vi "Perform Measurements.vi"(8 "error in":errorcluster, 9 "Measurement Context":refnum<class "Measure Call Context.lvclass">, 10 "Nominal output voltage":dbl, 11 "Reference values":T2) -> (0 "error out":errorcluster, 1 "Measurement Results":T1, 2 "Load out":refnum<k15>, 3 "Source out":refnum<k15>)   [LabVIEW 2021, in "Line Regulation_PMIC.lvlib"]
uses:
  Line Regulation_PMIC.lvlib
  Measurement Results.ctl
  <vilib>/Plug-In SDKs/Measurements/Measure Call Context/Measure Call Context.lvclass
  <vilib>/Plug-In SDKs/Measurements/Measure Call Context/Accessor/Is Canceled.vi
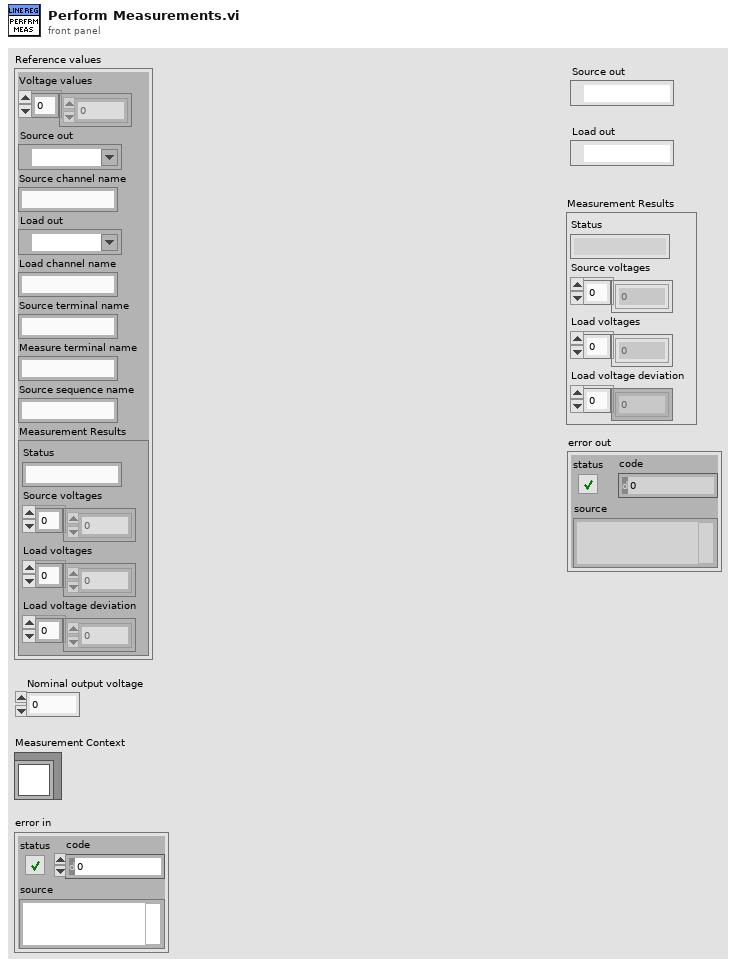
[diagram p1: front panel]
types:
  T1 = typedef "Line Regulation_PMIC.lvlib/Measurement Results.ctl" = cluster{"Status":string, "Source voltages":dbl[], "Load voltages":dbl[], "Load voltage deviation":dbl[]}
  T2 = cluster{"Voltage values":dbl[], "Source out":refnum<k15>, "Source channel name":string, "Load out":refnum<k15>, "Load channel name":string, "Source terminal name":string, "Measure terminal name":string, "Source sequence name":string, "Measurement Results":T1}
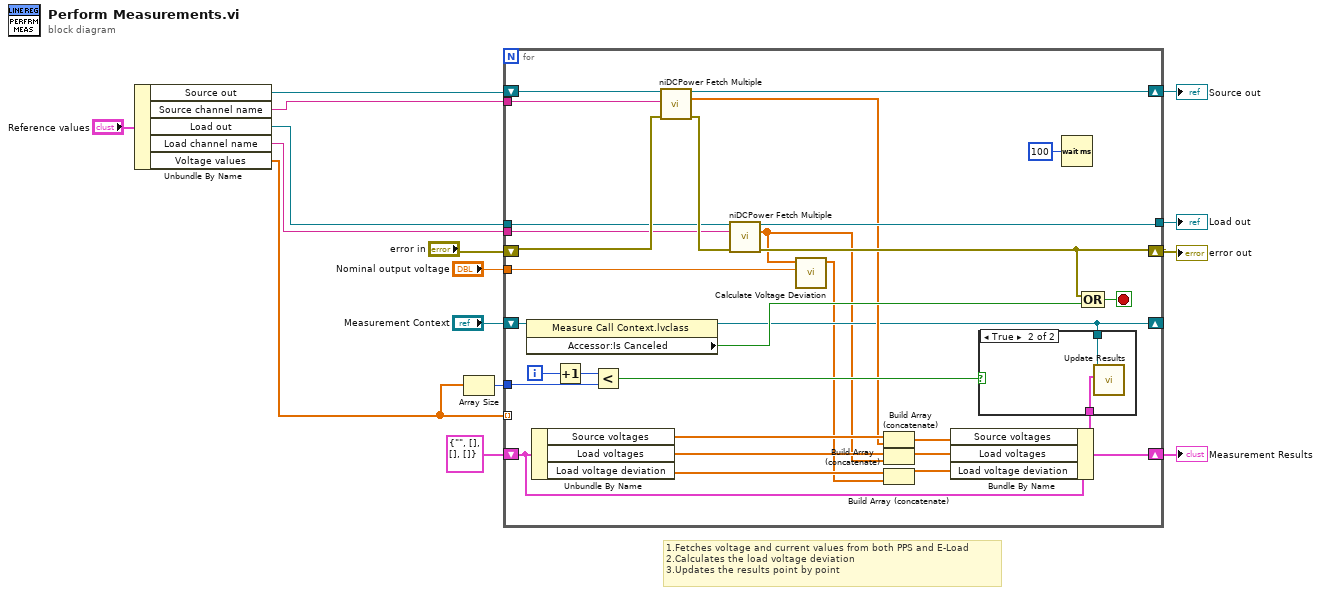
[diagram p0: block diagram]
diagram:
  # "1.Fetches voltage and current values from both PPS and E-Load\n2.Calculates the load voltage deviation\n3.Updates the results point by point"
  n1 = Unbundle By Name("Reference values") -> ("Source out"=w11:refnum<k15>, "Source channel name"=w10:string, "Load out"=w9:refnum<k15>, "Load channel name"=w8:string, "Voltage values"=w6:dbl[])
  n2 = Array Size(array=w6) -> (size(s)=w5:i32)
  n3 = for {
    shift-right: [w35] -> w14
    shift-left: "error in" -> [w41]
    shift-right: [w44] -> w4
    shift-left: w11 -> [w45]
    shift-right: [w31] -> w2
    shift-left: T1 {"Status"="", "Source voltages"=[], "Load voltages"=[], "Load voltage deviation"=[]} ("Measurement Results") -> [w32]
    tunnel: [w43] -> w3
    shift-right: [w26] -> _
    shift-left: "Measurement Context" -> [w27]
    tunnel: w10 -> [w25]
    tunnel: w9 -> [w24]
    tunnel: w8 -> [w23]
    tunnel: "Nominal output voltage" -> [w22]
    tunnel: w6 -> [_] mode=indexing
    tunnel: w5 -> [w17]
    i -> [w40]
    stop <- w36 stop-if-true
    n4 = property class="Measure Call Context.lvclass"(reference=w27) -> (reference out=w26:refnum<class "Measure Call Context.lvclass">, "Accessor:Is Canceled"=w37:bool)  [unwired: 1 in, 1 out]
    n5 = Unbundle By Name(w32) -> ("Source voltages"=w34:dbl[], "Load voltages"=w21:dbl[], "Load voltage deviation"=w19:dbl[])
    n6 = Increment(x=w40) -> (x+1=w39:i32)
    n7 = Less?(x=w39, y=w17) -> (x < y?=w38:bool)
    n8 = call <instrlib>:"niDCPower Fetch Multiple.vi"("instrument handle"=w45, "channel name"=w25, "error in (no error)"=w41) -> ("instrument handle out"=w44:refnum<k15>, "voltage measurements"=w30:dbl[], "error out"=w42:errorcluster)  [unwired: 2 in, 8 out]
    n9 = call <instrlib>:"niDCPower Fetch Multiple.vi"("instrument handle"=w24, "channel name"=w23, "error in (no error)"=w42) -> ("instrument handle out"=w43:refnum<k15>, "voltage measurements"=w20:dbl[], "error out"=w35:errorcluster)  [unwired: 2 in, 8 out]
    n10 = call "Calculate Voltage Deviation.vi"("Nominal output voltage"=w22, "Voltage measurements"=w20) -> ("Load voltage deviation"=w18:dbl[])  [unwired: 9 in]
    n11 = Build Array (concatenate)(w34, w30) -> (w33:dbl[])
    n12 = Build Array (concatenate)(w21, w20) -> (w29:dbl[])
    n13 = Build Array (concatenate)(w19, w18) -> (w28:dbl[])
    n14 = Bundle By Name(cluster=w32, "Source voltages"=w33, "Load voltages"=w29, "Load voltage deviation"=w28) -> (w31:T1)
    n15 = case shown="True" w38 {
      tunnel: w26 -> [_ w47]
      tunnel: w31 -> [_ w46]
      frame False {
      }
      frame True {
        n16 = call <vilib>:"Update Results.vi"("measurement results"=w46, "measure call context in"=w47) -> ()  [unwired: 8 in, 2 out]
      }
    }
    n17 = Wait (ms)(milliseconds to wait=u32 100) -> ()  [unwired: 1 out]
    n18 = Compound Arithmetic op=OR(w35, w37) -> (w36:bool)
  }
  "error out" <- w14
  "Source out" <- w4
  "Load out" <- w3
  "Measurement Results" <- w2
